vi "输入框.vi"(1 "提示信息":string) -> (0 "条形码输出":string)   [LabVIEW 2020]
uses:
  Global_Variable/Global.vi
panel:
  in  "字符串":string
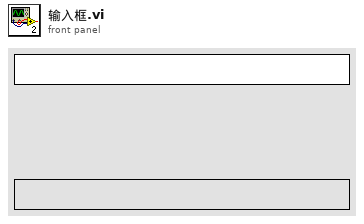
[diagram p1: front panel]
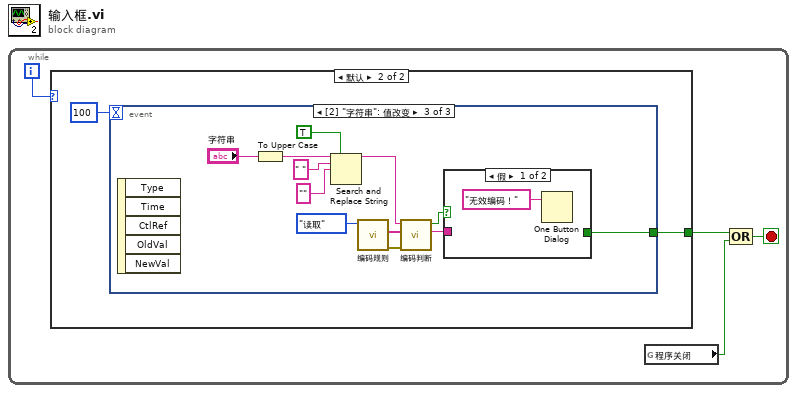
[diagram p0: block diagram]
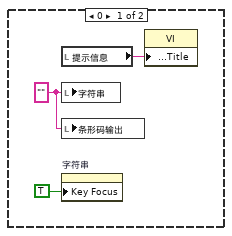
[diagram p2: hidden frame]
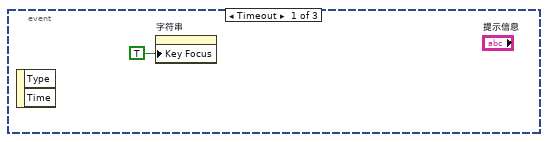
[diagram p3: hidden frame]
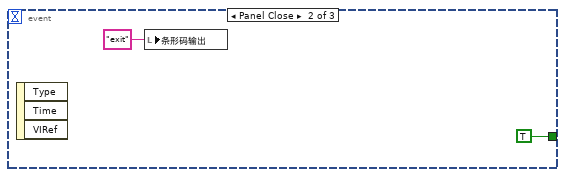
[diagram p4: hidden frame]
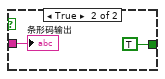
[diagram p5: hidden frame]
diagram:
  n1 = while {
    i -> [w3]
    stop <- w2 stop-if-true
    n2 = case shown="默认" w3 {
      tunnel: [_ w9] -> w4
      frame 0 {
        w7 = "" ("字符串")
        n3 = local read "提示信息"() -> (w6:string)
        n4 = local write "字符串"(w7) -> ()
        n5 = local write "条形码输出"(w7) -> ()
        n6 = property on="字符串" class="Str"("Key Focus"=TRUE ("键选中")) -> ()  [unwired: 2 in, 2 out]
        n7 = property class="VI"("Front Panel.Title"=w6) -> ()  [unwired: 2 in, 2 out]
      }
      frame Default {
        n8 = event shown="[2] \"字符串\": 值改变" {
          selector: _ -> [_ _ _]
          dyn-events: _ -> [_ _ _]
          timeout: 100 -> [_ _ _]
          tunnel: [_ TRUE w19] -> w9
          event Timeout {
            n9 = event-data() -> ()  [unwired: 1 in, 2 out]
            n10 = property on="字符串" class="Str"("Key Focus"=TRUE ("键选中")) -> ()  [unwired: 2 in, 2 out]
          }
          event Panel Close {
            n11 = event-data() -> ()  [unwired: 1 in, 3 out]
            n12 = local write "条形码输出"("exit" ("条形码输出")) -> ()
          }
          event "字符串": Value Change {
            n13 = event-data() -> ()  [unwired: 1 in, 5 out]
            n14 = To Upper Case(1:"字符串") -> (0:w18:string)
            n15 = Search and Replace String(replace all?=TRUE ("替换全部？(F)"), input string=w18, search string=" " ("搜索字符串"), replace string="" ("替换字符串(\"\")")) -> (result string=w13:string)  [unwired: 4 in, 3 out]
            n16 = call "编码规则.vi"("功能"=enum16{"读取", "写入"}."读取") -> ("错误输出"=w23:errorcluster, "正则表达式输出（多行）"=w24:string[])  [unwired: 8 in, 1 out]
            n17 = call "编码判断.vi"("错误输入"=w23, "编码规则"=w24, "输入编码"=w13) -> ("输出编码"=w21:string, "有效编码？"=w20:bool)  [unwired: 6 in, 1 out]
            n18 = case shown="假" w20 {
              tunnel: w21 -> [_ w27]
              tunnel: [_ TRUE] -> w19
              frame False {
                n19 = One Button Dialog(message="无效编码！" ("消息")) -> ()  [unwired: 1 in, 1 out]
              }
              frame True {
                "条形码输出" <- w27
              }
            }
          }
        }
      }
    }
    n20 = global read "Global.vi" "程序关闭"() -> (w1:bool)
    n21 = Compound Arithmetic op=OR ("复合运算")(w4, w1) -> (w2:bool)
  }
